vi "Get Templates.vi"(8 "Error In":errorcluster) -> (0 "Error Out":errorcluster, 2 "Circle Template":T1, 3 "Square Template":T1)   [LabVIEW 2018]
uses:
  <vilib>/vision/Image Controls.llb/IMAQ Image.ctl
  <vilib>/vision/Pattern Matching.llb/IMAQ Curve Parameters.ctl
  <vilib>/vision/NI_Vision_Development_Module.lvlib
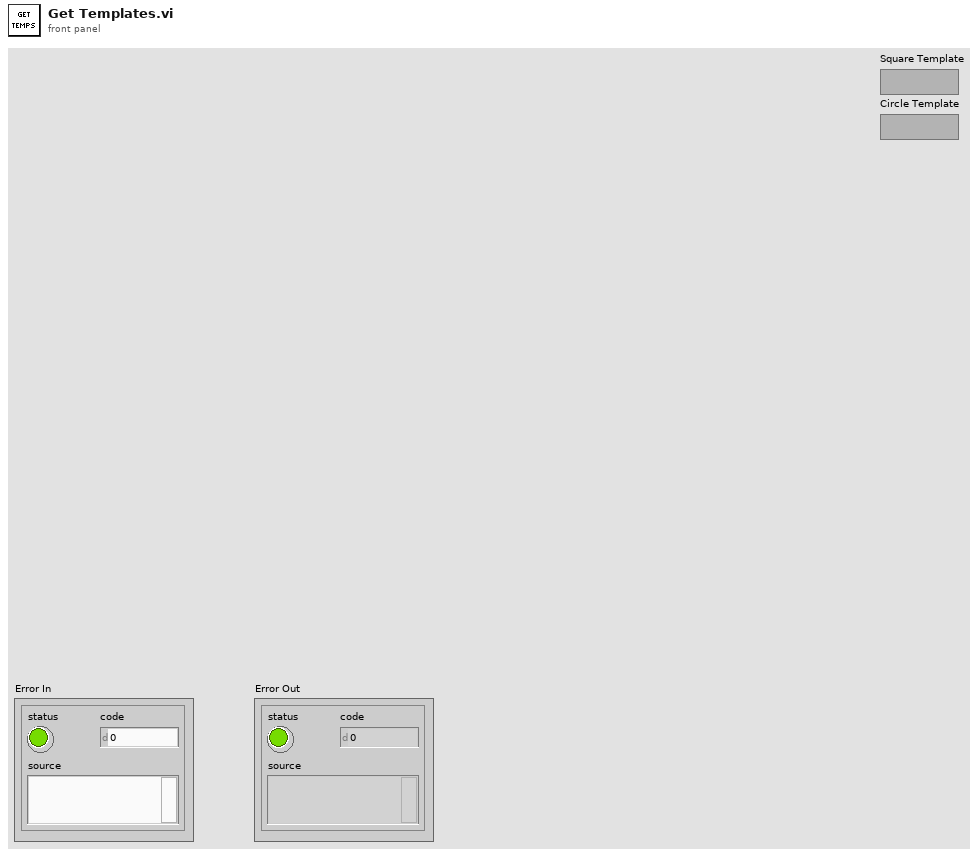
[diagram p1: front panel]
types:
  T1 = typedef "IMAQ Image.ctl" = refnum<image>
  T2 = typedef "IMAQ Curve Parameters.ctl" = cluster{"Extraction Mode":u32, "Edge Threshold":i32, "Edge Filter Size":u32, "Min Length":i32, "Row Search Step Size":i32, "Col Search Step Size":i32, "Max Endpoint Gap":i32, "Closed":bool, "Subpixel":bool}
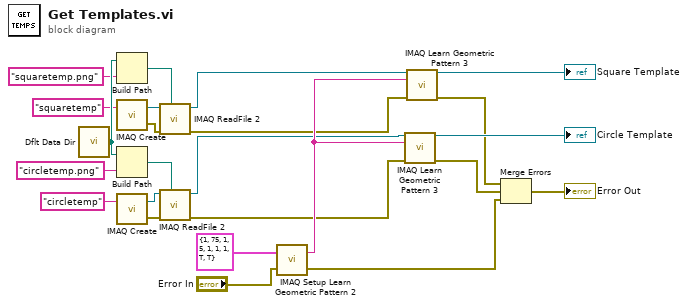
[diagram p0: block diagram]
diagram:
  n1 = call <vilib>:"Dflt Data Dir.vi"() -> ("App:Default Data Directory"=w21:path)
  n2 = Build Path(base path=w21, name or relative path="squaretemp.png") -> (appended path=w23:path)
  n3 = call "IMAQ Create"("Image Name"="squaretemp") -> ("New Image"=w16:T1, "error out"=w17:errorcluster)  [unwired: 4 in]
  n4 = Build Path(base path=w21, name or relative path="circletemp.png") -> (appended path=w24:path)
  n5 = call "IMAQ Create"("Image Name"="circletemp") -> ("New Image"=w18:T1, "error out"=w19:errorcluster)  [unwired: 4 in]
  n6 = call "IMAQ ReadFile 2"("File Path"=w23, "error in (no error)"=w17, "Image"=w16) -> ("error out"=w10:errorcluster, "Image Out"=w8:T1)  [unwired: 4 in, 3 out]
  n7 = call "IMAQ ReadFile 2"("File Path"=w24, "error in (no error)"=w19, "Image"=w18) -> ("error out"=w9:errorcluster, "Image Out"=w7:T1)  [unwired: 4 in, 3 out]
  n8 = call "IMAQ Setup Learn Geometric Pattern 2"("error in (no error)"="Error In", "Curve Parameters"=T2 {"Extraction Mode"=1, "Edge Threshold"=75, "Edge Filter Size"=1, "Min Length"=5, "Row Search Step Size"=1, "Col Search Step Size"=1, "Max Endpoint Gap"=1, "Closed"=TRUE, "Subpixel"=TRUE}) -> ("error out"=w1:errorcluster, "Learn Geometric Pattern 2 Setup Data"=w11:string)
  n9 = call "IMAQ Learn Geometric Pattern 3"("Template Image"=w7, "Learn Geometric Pattern 2 Setup Data"=w11, "error in (no error)"=w9) -> ("Template Image Out"=→"Circle Template":T1, "error out"=w2:errorcluster)  [unwired: 11 in]
  n10 = call "IMAQ Learn Geometric Pattern 3"("Template Image"=w8, "Learn Geometric Pattern 2 Setup Data"=w11, "error in (no error)"=w10) -> ("Template Image Out"=→"Square Template":T1, "error out"=w3:errorcluster)  [unwired: 11 in]
  n11 = Merge Errors(w3, w2, w1) -> (→"Error Out":errorcluster)
